vi "encoder.vi"(1 "Command input":T1={"Start meas"=33, "Command"="", "Length"=1, "Payload"=1} {"Start meas" max=1}) -> (0 "Command string":string)   [LabVIEW 2020]
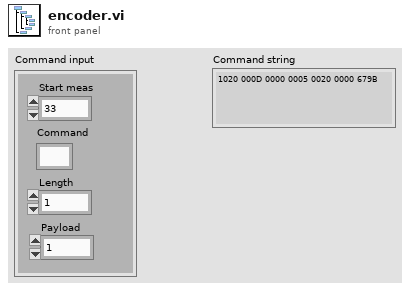
[diagram p1: front panel]
types:
  T1 = cluster{"Start meas":u8, "Command":string, "Length":u8, "Payload":u8}
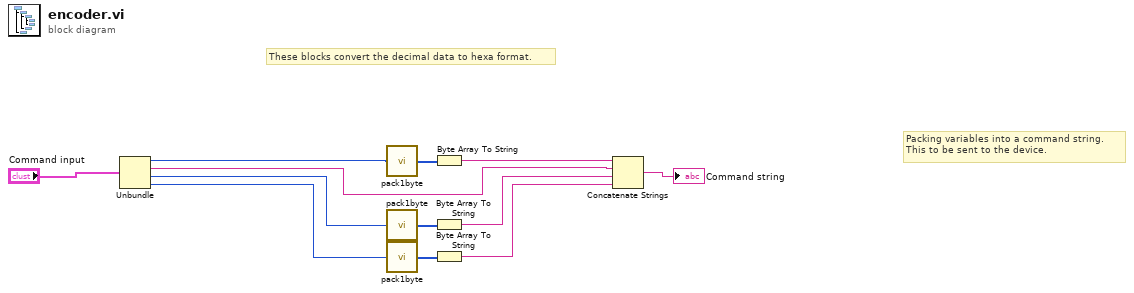
[diagram p0: block diagram]
diagram:
  # "These blocks convert the decimal data to hexa format."
  # "Packing variables into a command string.\nThis to be sent to the device."
  n1 = Unbundle("Command input") -> ("Start meas"=w9:u8, "Command"=w1:string, "Length"=w8:u8, "Payload"=w4:u8)
  n2 = call "pack1byte.vi"("Decimal In"=w9) -> ("Bytes out"=w10:u8[])
  n3 = call "pack1byte.vi"("Decimal In"=w8) -> ("Bytes out"=w7:u8[])
  n4 = call "pack1byte.vi"("Decimal In"=w4) -> ("Bytes out"=w5:u8[])
  n5 = Byte Array To String(unsigned byte array=w10) -> (string=w12:string)
  n6 = Byte Array To String(unsigned byte array=w7) -> (string=w6:string)
  n7 = Byte Array To String(unsigned byte array=w5) -> (string=w3:string)
  n8 = Concatenate Strings(w12, w1, w6, w3) -> (→"Command string":string)
